vi "Read String.vi"(8 "error in (no error)":errorcluster, 9 "element data type":string, 10 "Tag Name":string, 11 "Current Value Table in":refnum<class "Current Value Table.lvclass">) -> (0 "error out":errorcluster, 2 "value":string, 3 "Current Value Table out":refnum<class "Current Value Table.lvclass">)   [LabVIEW 2024, in "Current Value Table.lvlib" / "Current Value Table.lvclass"]
uses:
  Current Value Table.lvclass
  CVT_String/CVT_String.lvclass
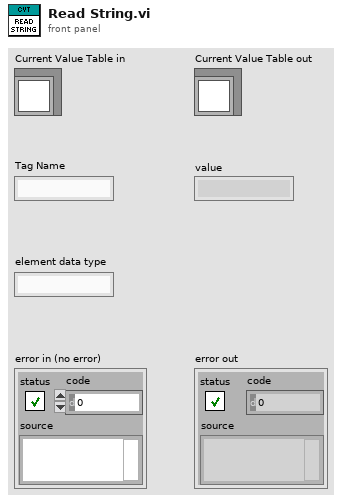
[diagram p1: front panel]
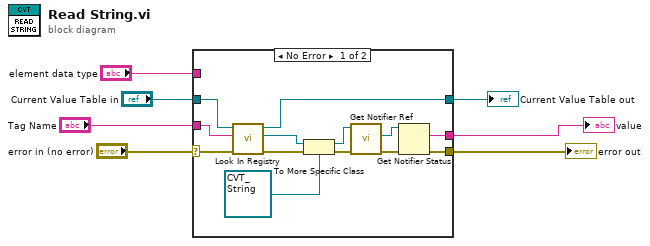
[diagram p0: block diagram]
diagram:
  n1 = case shown="No Error" "error in (no error)" {
    selector: "error in (no error)" -> [w9 w22]
    tunnel: [w11 w22] -> w6
    tunnel: [w8 w21] -> w4
    tunnel: "Current Value Table in" -> [w20 w21]
    tunnel: "element data type" -> [_ _]
    tunnel: "Tag Name" -> [w19 _]
    tunnel: [w14 _] -> w1
    frame No Error {
      n2 = call-dynamic "Look In Registry.vi"("error in (no error)"=w9, "Tag Name"=w19, "Current Value Table in"=w20) -> ("error out"=w10:errorcluster, "CVT_Item out"=w18:refnum<class "iCVT_Item.lvclass">, "Current Value Table out"=w8:refnum<class "Current Value Table.lvclass">)  [unwired: 5 in, 1 out]
      n3 = To More Specific Class(target class=refnum<class "CVT_String.lvclass"> refnum ("Current Value Table.lvlib:CVT_String.lvclass"), reference=w18, error in=w10) -> (specific class reference=w16:refnum<class "CVT_String.lvclass">, error out=w12:errorcluster)
      n4 = call-dynamic "Get Notifier Ref.vi"("error in (no error)"=w12, "CVT_String in"=w16) -> ("error out"=w13:errorcluster, "notifier out"=w15:refnum<notifier>)  [unwired: 7 in, 1 out]
      n5 = Get Notifier Status(notifier=w15, error in (no error)=w13) -> (current notification=w14:string, error out=w11:errorcluster)  [unwired: 3 out]
    }
    frame Error {
    }
  }
  "error out" <- w6
  "Current Value Table out" <- w4
  "value" <- w1
